vi "PXIe-4130_Reset.vi"(0 "User Reference":i32, 5 "error in (no error)":errorcluster) -> (19 "error out":errorcluster)   [LabVIEW 2018, in "PXIe-4130.lvclass"]
uses:
  PXIe-4130.lvclass
  Power_Supply Virtual/Power_Supply Virtual.lvclass
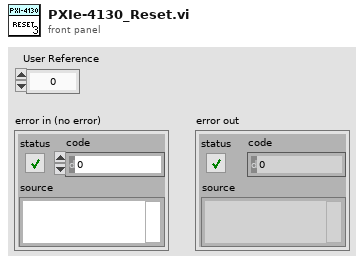
[diagram p1: front panel]
types:
  T1 = typedef "Class Attributes Cluster.ctl" = cluster{"Model Number":string, "Instrument Number":u8, "Rack ID":string, "Inst Mnemonic":string, "Comp Mnemonic":string, "Subsys Mnemonic":string, "IP Address":string, "Sub Address":string, "Firmware Rev":string, "Expected Options":string, "Required Options":string, "Excluded Options":string}
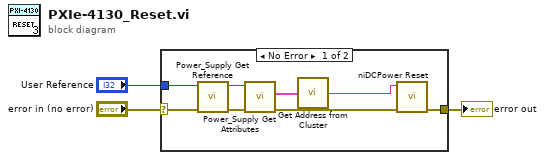
[diagram p0: block diagram]
diagram:
  n1 = case shown="No Error" "error in (no error)" {
    selector: "error in (no error)" -> [w9 w12]
    tunnel: [w6 w12] -> w2
    tunnel: "User Reference" -> [w8 _]
    frame No Error {
      n2 = call "Power_Supply Get Reference.vi"("error in (no error)"=w9, "Instrument Reference"=w8) -> ("error out"=w11:errorcluster, "Power_Supply Virtual.lvclass"=w10:refnum<class "Power_Supply Virtual.lvclass">)  [unwired: 7 in, 1 out]
      n3 = call-dynamic "Power_Supply Get Attributes.vi"("error in (no error)"=w11, "Power_Supply Virtual in"=w10) -> ("error out"=w7:errorcluster, "Class Attributes"=w5:T1)  [unwired: 7 in, 1 out]
      n4 = call "Get Address from Cluster.vi"("Class Attributes"=w5) -> ("Address"=w4:string)  [unwired: 4 in]
      n5 = call <instrlib>:"niDCPower Reset.vi"("error in (no error)"=w7, "instrument handle"=w4) -> ("error out"=w6:errorcluster)  [unwired: 8 in, 1 out]
    }
    frame Error {
    }
  }
  "error out" <- w2
